vi "nc_inq_varndims.vi"(4 "varid":i32, 5 "NC":T1) -> (1 "ndims":i32)   [LabVIEW 2016]
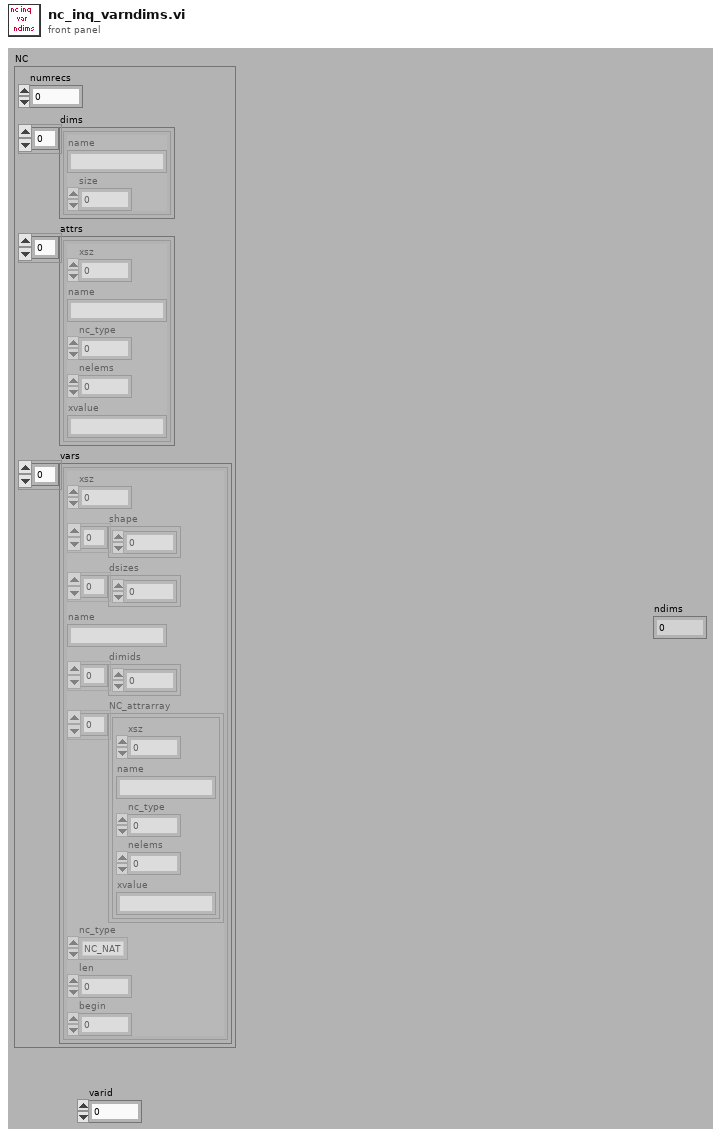
[diagram p1: front panel]
types:
  T1 = cluster{"numrecs":u64, "dims":cluster{"name":string, "size":u64}[], "attrs":cluster{"xsz":u64, "name":string, "nc_type":u16, "nelems":u64, "xvalue":string}[], "vars":cluster{"xsz":u64, "shape":u64[], "dsizes":u64[], "name":string, "dimids":u64[], "NC_attrarray":cluster{"xsz":u64, "name":string, "nc_type":u16, "nelems":u64, "xvalue":string}[], "nc_type":enum16{"NC_NAT", "NC_BYTE", "NC_CHAR", "NC_SHORT", "NC_INT", "NC_FLOAT", "NC_DOUBLE"}, "len":u64, "begin":u64}[]}
  T2 = cluster{"xsz":u64, "shape":u64[], "dsizes":u64[], "name":string, "dimids":u64[], "NC_attrarray":cluster{"xsz":u64, "name":string, "nc_type":u16, "nelems":u64, "xvalue":string}[], "nc_type":enum16{"NC_NAT", "NC_BYTE", "NC_CHAR", "NC_SHORT", "NC_INT", "NC_FLOAT", "NC_DOUBLE"}, "len":u64, "begin":u64}[]
  T3 = cluster{"xsz":u64, "shape":u64[], "dsizes":u64[], "name":string, "dimids":u64[], "NC_attrarray":cluster{"xsz":u64, "name":string, "nc_type":u16, "nelems":u64, "xvalue":string}[], "nc_type":enum16{"NC_NAT", "NC_BYTE", "NC_CHAR", "NC_SHORT", "NC_INT", "NC_FLOAT", "NC_DOUBLE"}, "len":u64, "begin":u64}
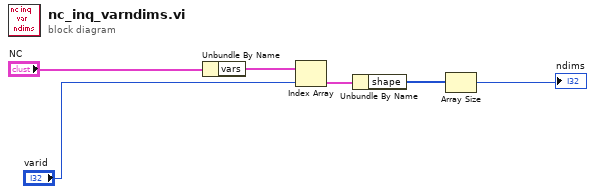
[diagram p0: block diagram]
diagram:
  n1 = Unbundle By Name("NC") -> ("vars"=w3:T2)
  n2 = Index Array(array=w3, index="varid") -> (element=w4:T3)
  n3 = Unbundle By Name(w4) -> ("shape"=w5:u64[])
  n4 = Array Size(array=w5) -> (size(s)=→"ndims":i32)
